vi "updateTestLog.vi"(8 "error in (no error)":errorcluster, 11 "Model in":refnum<class "Model.lvclass">) -> (0 "error out":errorcluster, 3 "Model out":refnum<class "Model.lvclass">)   [LabVIEW 2013, in "Model.lvclass"]
uses:
  Model.lvclass
  Model.lvclass/Model.ctl
  UserEvents/UserEvents.lvclass/UserEvents.ctl
  ApplicationElements/Log/TestDataLog/TestDataLog.lvclass
  <userlib>/Common/Log/Log/Log.lvclass
  UserEvents/UserEvents.lvclass
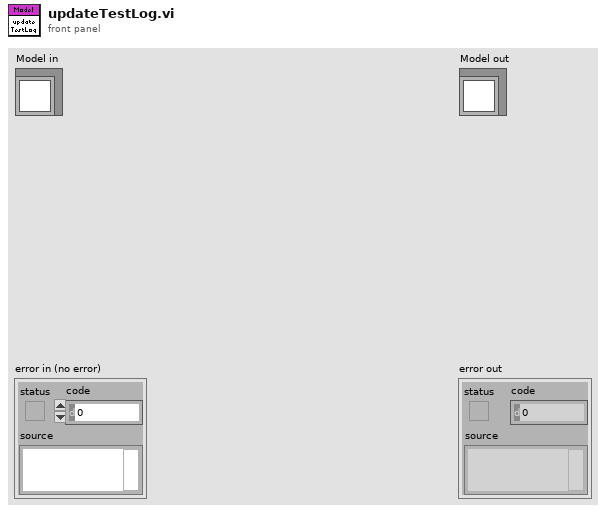
[diagram p1: front panel]
types:
  T1 = typedef "M2AADTTypedefs.lvlib/PubDataEvents.ctl" = cluster{"State":refnum<user-event>, "ErrorCode":refnum<user-event>, "OutputData":refnum<user-event>, "InputData":refnum<user-event>, "ControllerData":refnum<user-event>, "TestStatus":refnum<user-event>, "LogPath":refnum<user-event>, "StiffnessData":refnum<user-event>}
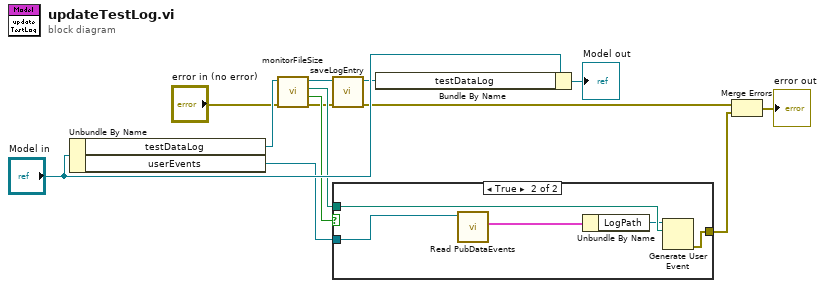
[diagram p0: block diagram]
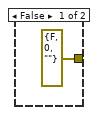
[diagram p2: hidden frame]
diagram:
  n1 = Unbundle By Name("Model in") -> ("testDataLog"=w9:refnum<class "TestDataLog.lvclass">, "userEvents"=w1:refnum<class "UserEvents.lvclass">)
  n2 = call <userlib>:"monitorFileSize.vi"("error in (no error)"="error in (no error)", "Logger in"=w9) -> ("error out"=w5:errorcluster, "newValue?"=w7:bool, "logFilePath"=w6:path, "Logger out"=w10:refnum<class "TestDataLog.lvclass">)  [unwired: 6 in]
  n3 = call-dynamic "saveLogEntry.vi"("error in (no error)"=w5, "Logger in"=w10) -> ("error out"=w4:errorcluster, "Logger out"=w11:refnum<class "TestDataLog.lvclass">)  [unwired: 8 in]
  n4 = case shown="True" w7 {
    tunnel: w6 -> [_ w19]
    tunnel: [errorcluster {"status"=FALSE, "code"=0, "source"=""} ("error out") w18] -> w3
    tunnel: w1 -> [_ w15]
    frame False {
    }
    frame True {
      n5 = call "Read PubDataEvents.vi"("UserEvents in"=w15) -> ("PubDataEvents"=w17:T1)  [unwired: 9 in, 1 out]
      n6 = Unbundle By Name(w17) -> ("LogPath"=w16:refnum<user-event>)
      n7 = Generate User Event(user event=w16, event data cluster=w19) -> (error out=w18:errorcluster)  [unwired: 2 in, 1 out]
    }
  }
  n8 = Bundle By Name(cluster="Model in", "testDataLog"=w11) -> (→"Model out":refnum<class "Model.lvclass">)
  n9 = Merge Errors(w4, w3) -> (→"error out":errorcluster)
